vi "HIOKI PW3390 Conf Measure Item.vi"(0 "VISA Resource":refnum<visa-resource-name>, 1 "Power":T5, 2 "Power Sum":T4, 3 "Integrate":T6, 4 "U":T1, 5 "I":T1, 7 "error in (no error)":errorcluster, 8 "Set/Query (F: Set)":bool, 9 "Efficiency":T8, 10 "All Clear (F: Off)":bool, 11 "Option":T7, 13 "OPC query (T: ON)":bool=TRUE, 15 "Error Out (F: Off)":bool) -> (17 "Option out":cluster{bool, bool, bool, bool}, 19 "Efficiency out":T3, 20 "VISA Resource out":refnum<visa-resource-name>, 21 "Power out":cluster{bool, bool, bool, bool}[](array[cluster]), 22 "Power Sum out":cluster{bool, bool, bool}[](array[cluster]), 23 "Integrate out":cluster{bool, bool, bool, bool}[](array[cluster]), 24 "U out":T2(array[cluster]), 25 "I out":T2(array[cluster]), 27 "error out":errorcluster)   [LabVIEW 2009]
doc: "Set/Query\n Set: Send the setting commands for the device.\n Query: Query the setting of the device.\n\nAll Clear\n Initializes the Output data items.\n All output data items become OFF.\n\nPower\n Sets the normal measurement output items of the various channels.\n\nPower Sum\n Sets the normal measurement output items of SUM.\n\nU\n Sets the voltage data output items.\n\nI\n Sets the current data output items.\n\nIntegrate\n Sets the Integration data output items.\n\nEfficiency\n Sets the output items of the efficiency/loss calculation formula.\n\nOption\n Sets the output items of Option."
panel:
  # "P"
  # "P"
  # "S"
  # "S"
  # "Q"
  # "Q"
  # "PF"
  # "PF"
  # "DEG"
  # "DEG"
  # "FREQ"
  # "CH1"
  # "CH2"
  # "CH3"
  # "CH4"
  # "SUM12"
  # "SUM34"
  # "SUM123"
  # "CH1"
  # "CH2"
  # "CH3"
  # "CH4"
  # "SUM12"
  # "SUM34"
  # "SUM123"
  # "IH+"
  # "IH-"
  # "IH"
  # "WP+"
  # "WP-"
  # "WP"
  # "WP+ SUM"
  # "WP- SUM"
  # "WP SUM"
  # "Elapsed time"
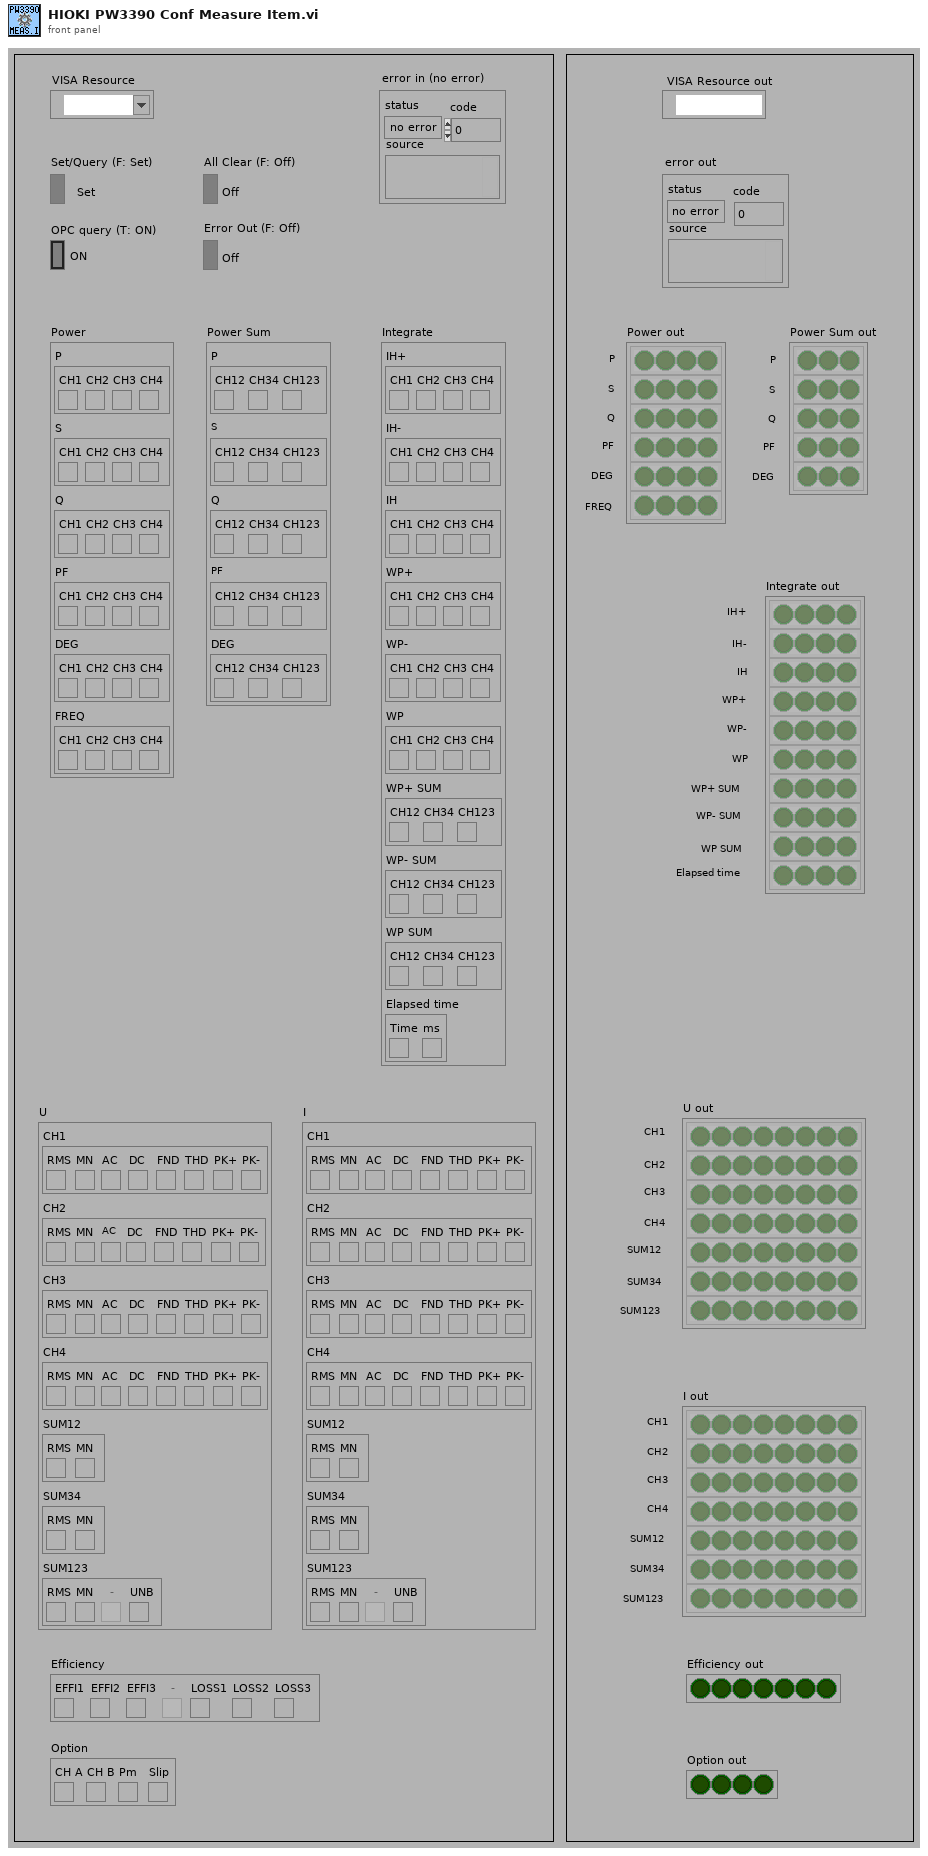
[diagram p1: front panel]
types:
  T1 = cluster{"CH1":cluster{"RMS":bool, "MN ":bool, "AC  ":bool, "DC  ":bool, "FND":bool, "THD":bool, "PK+":bool, "PK-":bool}, "CH2":cluster{"RMS":bool, "MN ":bool, "AC  ":bool, "DC  ":bool, "FND":bool, "THD":bool, "PK+":bool, "PK-":bool}, "CH3":cluster{"RMS":bool, "MN ":bool, "AC  ":bool, "DC  ":bool, "FND":bool, "THD":bool, "PK+":bool, "PK-":bool}, "CH4":cluster{"RMS":bool, "MN ":bool, "AC  ":bool, "DC  ":bool, "FND":bool, "THD":bool, "PK+":bool, "PK-":bool}, "SUM12":cluster{"RMS":bool, "MN ":bool}, "SUM34":cluster{"RMS":bool, "MN ":bool}, "SUM123":cluster{"RMS":bool, "MN ":bool, "  -   ":bool, "UNB":bool}}
  T2 = cluster{bool, bool, bool, bool, bool, bool, bool, bool}[]
  T3 = cluster{bool, bool, bool, bool, bool, bool, bool}
  T4 = cluster{"P":cluster{"CH12":bool, "CH34":bool, "CH123":bool}, "S":cluster{"CH12":bool, "CH34":bool, "CH123":bool}, "Q":cluster{"CH12":bool, "CH34":bool, "CH123":bool}, "PF":cluster{"CH12":bool, "CH34":bool, "CH123":bool}, "DEG":cluster{"CH12":bool, "CH34":bool, "CH123":bool}}
  T5 = cluster{"P":cluster{"CH1":bool, "CH2":bool, "CH3":bool, "CH4":bool}, "S":cluster{"CH1":bool, "CH2":bool, "CH3":bool, "CH4":bool}, "Q":cluster{"CH1":bool, "CH2":bool, "CH3":bool, "CH4":bool}, "PF":cluster{"CH1":bool, "CH2":bool, "CH3":bool, "CH4":bool}, "DEG":cluster{"CH1":bool, "CH2":bool, "CH3":bool, "CH4":bool}, "FREQ":cluster{"CH1":bool, "CH2":bool, "CH3":bool, "CH4":bool}}
  T6 = cluster{"IH+":cluster{"CH1":bool, "CH2":bool, "CH3":bool, "CH4":bool}, "IH-":cluster{"CH1":bool, "CH2":bool, "CH3":bool, "CH4":bool}, "IH":cluster{"CH1":bool, "CH2":bool, "CH3":bool, "CH4":bool}, "WP+":cluster{"CH1":bool, "CH2":bool, "CH3":bool, "CH4":bool}, "WP-":cluster{"CH1":bool, "CH2":bool, "CH3":bool, "CH4":bool}, "WP":cluster{"CH1":bool, "CH2":bool, "CH3":bool, "CH4":bool}, "WP+ SUM":cluster{"CH12":bool, "CH34":bool, "CH123":bool}, "WP- SUM":cluster{"CH12":bool, "CH34":bool, "CH123":bool}, "WP SUM":cluster{"CH12":bool, "CH34":bool, "CH123":bool}, "Elapsed time":cluster{"Time":bool, "ms":bool}}
  T7 = cluster{"CH A":bool, "CH B":bool, "Pm  ":bool, "Slip":bool}
  T8 = cluster{"EFFI1":bool, "EFFI2":bool, "EFFI3":bool, "  -   ":bool, "LOSS1":bool, "LOSS2":bool, "LOSS3":bool}
  T9 = cluster{"Boolean array[0]":bool, "Boolean array[1]":bool, "Boolean array[2]":bool}
  T10 = cluster{"Boolean array[0]":bool, "Boolean array[1]":bool, "Boolean array[2]":bool, "Boolean array[3]":bool}
  T11 = cluster{"Boolean array[0]":bool, "Boolean array[1]":bool, "Boolean array[2]":bool, "Boolean array[3]":bool, "Boolean array[4]":bool, "Boolean array[5]":bool, "Boolean array[6]":bool, "Boolean array[7]":bool}
  T12 = cluster{"Boolean array[0]":bool, "Boolean array[1]":bool, "Boolean array[2]":bool, "Boolean array[3]":bool, "Boolean array[4]":bool, "Boolean array[5]":bool, "Boolean array[6]":bool}
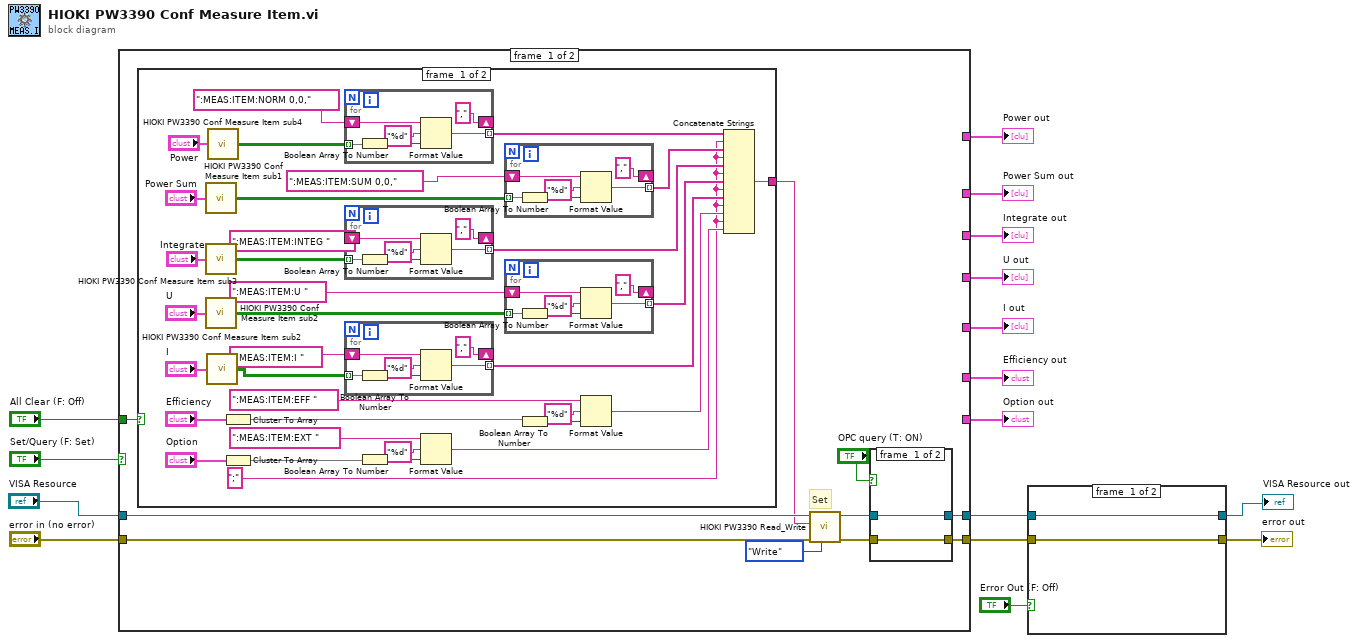
[diagram p0: block diagram]
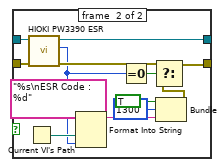
[diagram p2: hidden frame]
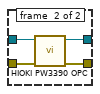
[diagram p3: hidden frame]
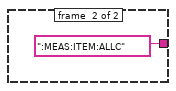
[diagram p4: hidden frame]
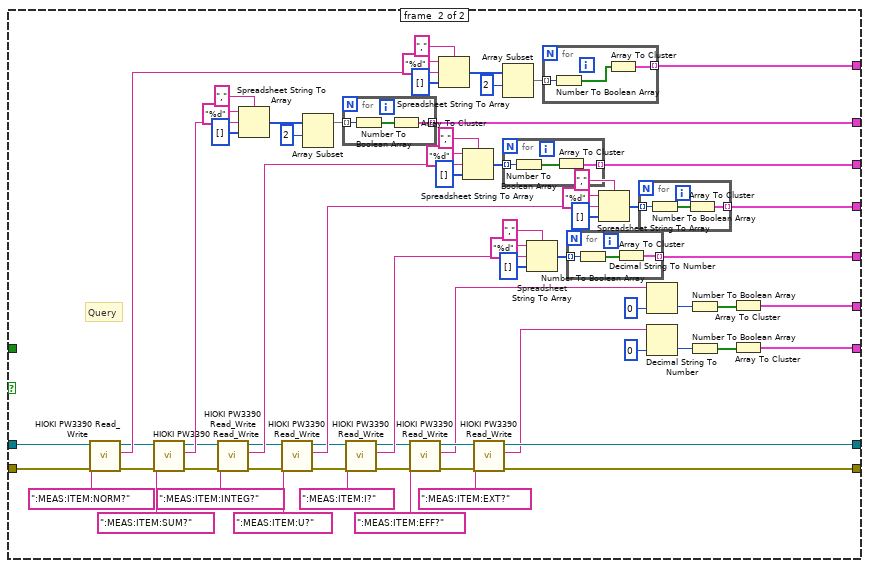
[diagram p5: hidden frame]
diagram:
  n1 = case shown="FALSE" "Set/Query (F: Set)" {
    tunnel: "error in (no error)" -> [w25 w163]
    tunnel: [w17 w127] -> w13
    tunnel: "VISA Resource" -> [w26 w164]
    tunnel: [w18 w128] -> w12
    tunnel: [_ w132] -> w6
    tunnel: [_ w131] -> w5
    tunnel: [_ w130] -> w4
    tunnel: [_ w129] -> w3
    tunnel: [_ w98] -> w1
    tunnel: [_ w100] -> w2
    tunnel: "All Clear (F: Off)" -> [w22 _]
    tunnel: [_ w102] -> w7
    frame #0 {
      # "Set"
      n2 = case shown="FALSE" w22 {
        tunnel: [w47 ":MEAS:ITEM:ALLC"] -> w23
        frame #0 {
          w48 = ";"
          n3 = call <instrlib>:"HIOKI PW3390 Conf Measure Item sub1.vi"("Power Sum"="Power Sum") -> ("Power Sum out"=w34:bool[][])
          n4 = call <instrlib>:"HIOKI PW3390 Conf Measure Item sub3.vi"("Integrate"="Integrate") -> ("Integrate out"=w44:bool[][])
          n5 = call <instrlib>:"HIOKI PW3390 Conf Measure Item sub2.vi"("U or I"="U") -> ("U or I out"=w46:bool[][])
          n6 = call <instrlib>:"HIOKI PW3390 Conf Measure Item sub2.vi"("U or I"="I") -> ("U or I out"=w45:bool[][])
          n7 = call <instrlib>:"HIOKI PW3390 Conf Measure Item sub4.vi"("Power"="Power") -> ("Power out"=w36:bool[][])
          n8 = Cluster To Array(cluster="Efficiency") -> (array=w42:bool[])
          n9 = Cluster To Array(cluster="Option") -> (array=w40:bool[])
          n10 = for {
            shift-right: [","] -> _
            shift-left: ":MEAS:ITEM:NORM 0,0," -> [w68]
            tunnel: [w69] -> w51 mode=indexing
            tunnel: w36 -> [w67] mode=indexing
            n11 = Boolean Array To Number(Boolean array=w67) -> (number=w71:u32)
            n12 = Format Value(string ("")=w68, format string="%d" ("形式文字列"), value (0)=w71) -> (output string=w69:string)
          }
          n13 = for {
            shift-right: [","] -> _
            shift-left: ":MEAS:ITEM:INTEG " -> [w86]
            tunnel: [w87] -> w49 mode=indexing
            tunnel: w44 -> [w85] mode=indexing
            n14 = Boolean Array To Number(Boolean array=w85) -> (number=w89:u32)
            n15 = Format Value(string ("")=w86, format string="%d" ("形式文字列"), value (0)=w89) -> (output string=w87:string)
          }
          n16 = for {
            shift-right: [","] -> _
            shift-left: ":MEAS:ITEM:I " -> [w92]
            tunnel: [w93] -> w60 mode=indexing
            tunnel: w45 -> [w91] mode=indexing
            n17 = Boolean Array To Number(Boolean array=w91) -> (number=w95:u32)
            n18 = Format Value(string ("")=w92, format string="%d" ("形式文字列"), value (0)=w95) -> (output string=w93:string)
          }
          n19 = Boolean Array To Number(Boolean array=w40) -> (number=w63:u32)
          n20 = Format Value(string ("")=":MEAS:ITEM:EXT ", format string="%d" ("形式文字列"), value (0)=w63) -> (output string=w62:string)
          n21 = for {
            shift-right: [","] -> _
            shift-left: ":MEAS:ITEM:SUM 0,0," -> [w74]
            tunnel: [w75] -> w50 mode=indexing
            tunnel: w34 -> [w73] mode=indexing
            n22 = Boolean Array To Number(Boolean array=w73) -> (number=w77:u32)
            n23 = Format Value(string ("")=w74, format string="%d" ("形式文字列"), value (0)=w77) -> (output string=w75:string)
          }
          n24 = for {
            shift-right: [","] -> _
            shift-left: ":MEAS:ITEM:U " -> [w80]
            tunnel: [w81] -> w59 mode=indexing
            tunnel: w46 -> [w79] mode=indexing
            n25 = Boolean Array To Number(Boolean array=w79) -> (number=w83:u32)
            n26 = Format Value(string ("")=w80, format string="%d" ("形式文字列"), value (0)=w83) -> (output string=w81:string)
          }
          n27 = Boolean Array To Number(Boolean array=w42) -> (number=w65:u32)
          n28 = Format Value(string ("")=":MEAS:ITEM:EFF ", format string="%d" ("形式文字列"), value (0)=w65) -> (output string=w61:string)
          n29 = Concatenate Strings(w51, w48, w50, w48, w49, w48, w59, w48, w60, w48, w61, w48, w62) -> (w47:string)
        }
        frame #1 {
        }
      }
      n30 = call <instrlib>:"HIOKI PW3390 Read_Write.vi"("Read/Write"=enum16{"Read", "Write"}."Write", "error in (no error)"=w25, "data in"=w23, "VISA Resource"=w26) -> ("error out"=w19:errorcluster, "VISA Resource out"=w20:refnum<visa-resource-name>)  [unwired: 5 in, 1 out]
      n31 = case shown="TRUE" "OPC query (T: ON)" {
        tunnel: [w28 w32] -> w18
        tunnel: [w27 w31] -> w17
        tunnel: w20 -> [w28 w30]
        tunnel: w19 -> [w27 w29]
        frame #0 {
        }
        frame #1 {
          n32 = call <instrlib>:"HIOKI PW3390 OPC.vi"("error in (no error)"=w29, "VISA Resource"=w30) -> ("error out"=w31:errorcluster, "VISA Resource out"=w32:refnum<visa-resource-name>)  [unwired: 7 in, 1 out]
        }
      }
    }
    frame #1 {
      # "Query"
      n33 = call <instrlib>:"HIOKI PW3390 Read_Write.vi"("error in (no error)"=w163, "data in"=":MEAS:ITEM:NORM?", "VISA Resource"=w164) -> ("error out"=w115:errorcluster, "data out"=w160:string, "VISA Resource out"=w116:refnum<visa-resource-name>)  [unwired: 6 in]
      n34 = call <instrlib>:"HIOKI PW3390 Read_Write.vi"("error in (no error)"=w115, "data in"=":MEAS:ITEM:SUM?", "VISA Resource"=w116) -> ("error out"=w118:errorcluster, "data out"=w136:string, "VISA Resource out"=w117:refnum<visa-resource-name>)  [unwired: 6 in]
      n35 = call <instrlib>:"HIOKI PW3390 Read_Write.vi"("error in (no error)"=w118, "data in"=":MEAS:ITEM:INTEG?", "VISA Resource"=w117) -> ("error out"=w119:errorcluster, "data out"=w135:string, "VISA Resource out"=w120:refnum<visa-resource-name>)  [unwired: 6 in]
      n36 = Spreadsheet String To Array(delimiter (Tab)="," ("デリミタ（Tab）"), format string="%d" ("形式文字列"), spreadsheet string=w136, array type (2D Dbl)=u8[] []) -> (array=w105:u8[])
      n37 = call <instrlib>:"HIOKI PW3390 Read_Write.vi"("error in (no error)"=w119, "data in"=":MEAS:ITEM:U?", "VISA Resource"=w120) -> ("error out"=w122:errorcluster, "data out"=w134:string, "VISA Resource out"=w121:refnum<visa-resource-name>)  [unwired: 6 in]
      n38 = Array Subset(array=w105, index=2 ("指標")) -> (w106:u8[])  [unwired: 1 in]
      n39 = for {
        tunnel: w106 -> [w176] mode=indexing
        tunnel: [w174] -> w132 mode=indexing
        n40 = Number To Boolean Array(number=w176) -> (Boolean array=w175:bool[])
        n41 = Array To Cluster(array=w175) -> (cluster=w174:T9)
      }
      n42 = call <instrlib>:"HIOKI PW3390 Read_Write.vi"("error in (no error)"=w122, "data in"=":MEAS:ITEM:I?", "VISA Resource"=w121) -> ("error out"=w123:errorcluster, "data out"=w133:string, "VISA Resource out"=w124:refnum<visa-resource-name>)  [unwired: 6 in]
      n43 = call <instrlib>:"HIOKI PW3390 Read_Write.vi"("error in (no error)"=w123, "data in"=":MEAS:ITEM:EFF?", "VISA Resource"=w124) -> ("error out"=w126:errorcluster, "data out"=w112:string, "VISA Resource out"=w125:refnum<visa-resource-name>)  [unwired: 6 in]
      n44 = Spreadsheet String To Array(delimiter (Tab)="," ("デリミタ（Tab）"), format string="%d" ("形式文字列"), spreadsheet string=w160, array type (2D Dbl)=u8[] []) -> (array=w107:u8[])
      n45 = Spreadsheet String To Array(delimiter (Tab)="," ("デリミタ（Tab）"), format string="%d" ("形式文字列"), spreadsheet string=w135, array type (2D Dbl)=u8[] []) -> (array=w144:u8[])
      n46 = call <instrlib>:"HIOKI PW3390 Read_Write.vi"("error in (no error)"=w126, "data in"=":MEAS:ITEM:EXT?", "VISA Resource"=w125) -> ("error out"=w127:errorcluster, "data out"=w113:string, "VISA Resource out"=w128:refnum<visa-resource-name>)  [unwired: 6 in]
      n47 = Array Subset(array=w107, index=2 ("指標")) -> (w108:u8[])  [unwired: 1 in]
      n48 = for {
        tunnel: w144 -> [w170] mode=indexing
        tunnel: [w168] -> w131 mode=indexing
        n49 = Number To Boolean Array(number=w170) -> (Boolean array=w169:bool[])
        n50 = Array To Cluster(array=w169) -> (cluster=w168:T10)
      }
      n51 = Spreadsheet String To Array(delimiter (Tab)="," ("デリミタ（Tab）"), format string="%d" ("形式文字列"), spreadsheet string=w133, array type (2D Dbl)=u8[] []) -> (array=w137:u8[])
      n52 = for {
        tunnel: w108 -> [w179] mode=indexing
        tunnel: [w177] -> w102 mode=indexing
        n53 = Number To Boolean Array(number=w179) -> (Boolean array=w178:bool[])
        n54 = Array To Cluster(array=w178) -> (cluster=w177:T10)
      }
      n55 = for {
        tunnel: w137 -> [w167] mode=indexing
        tunnel: [w165] -> w129 mode=indexing
        n56 = Number To Boolean Array(number=w167) -> (Boolean array=w166:bool[])
        n57 = Array To Cluster(array=w166) -> (cluster=w165:T11)
      }
      n58 = Spreadsheet String To Array(delimiter (Tab)="," ("デリミタ（Tab）"), format string="%d" ("形式文字列"), spreadsheet string=w134, array type (2D Dbl)=u8[] []) -> (array=w145:u8[])
      n59 = for {
        tunnel: w145 -> [w173] mode=indexing
        tunnel: [w171] -> w130 mode=indexing
        n60 = Number To Boolean Array(number=w173) -> (Boolean array=w172:bool[])
        n61 = Array To Cluster(array=w172) -> (cluster=w171:T11)
      }
      n62 = Decimal String To Number(string=w112, default (0L)=u8 0) -> (number=w111:u8)  [unwired: 1 in, 1 out]
      n63 = Decimal String To Number(string=w113, default (0L)=u8 0) -> (number=w114:u8)  [unwired: 1 in, 1 out]
      n64 = Number To Boolean Array(number=w111) -> (Boolean array=w101:bool[])
      n65 = Number To Boolean Array(number=w114) -> (Boolean array=w99:bool[])
      n66 = Array To Cluster(array=w101) -> (cluster=w100:T12)
      n67 = Array To Cluster(array=w99) -> (cluster=w98:T10)
    }
  }
  "Power out" <- w7
  "Power Sum out" <- w6
  "Integrate out" <- w5
  "U out" <- w4
  "I out" <- w3
  "Efficiency out" <- w2
  "Option out" <- w1
  n68 = case shown="TRUE" "Error Out (F: Off)" {
    tunnel: w12 -> [w181 w194]
    tunnel: w13 -> [w180 w193]
    tunnel: [w180 w183] -> w11
    tunnel: [w181 w192] -> w8
    frame #0 {
    }
    frame #1 {
      n69 = Current VI's Path() -> (path=w190:path)
      n70 = call <instrlib>:"HIOKI PW3390 ESR.vi"("error in (no error)"=w193, "VISA Resource"=w194) -> ("error out"=w184:errorcluster, "Output Value"=w182:u8, "VISA Resource out"=w192:refnum<visa-resource-name>)  [unwired: 6 in, 1 out]
      n71 = Format Into String(format string="%s\nESR Code : %d", w190, w182) -> (resulting string=w186:string)  [unwired: 2 in, 1 out]
      n72 = Equal To 0?(x=w182) -> (x = 0?=w191:bool)
      n73 = Bundle("status"=TRUE, "code"=1300, w186) -> (w185:cluster{"status":bool, "code":i32, string})  [unwired: 1 in]
      n74 = Select(t=w184, s=w191, f=w185) -> (s? t:f=w183:errorcluster)
    }
  }
  "error out" <- w11
  "VISA Resource out" <- w8
